vi "Load Config.vi"(8 "error in (no error)":errorcluster, 11 "CurrentInChannel in":refnum<class "CurrentInChannel.lvclass">) -> (0 "error out":errorcluster, 3 "CurrentInChannel out":refnum<class "CurrentInChannel.lvclass">)   [LabVIEW 2020, in "VolatusDAQConfig.lvlib" / "CurrentInChannel.lvclass"]
uses:
  CurrentInChannel.lvclass
  CurrentInChannel.lvclass/CurrentInChannel.ctl
  VolatusConfig/VolatusConfigElement/VolatusConfigElement.lvclass
  lv-cdm/CDM-Config/Config Element/Config Element.lvclass
  C:/dev/lv20CE/relink/lv-volatus/VolatusDAQConfig/DAQmxChannel/DAQmxChannel.lvclass
  C:/dev/lv20CE/relink/lv-volatus/VolatusConfig/Channel/Channel Config.lvclass
  C:/dev/lv20CE/relink/lv-volatus/VolatusConfig/VolatusConfigElement/VolatusConfigElement.lvclass
  C:/dev/lv20CE/relink/lv-volatus/VolatusDAQConfig/CurrentInChannel/CurrentInChannel.lvclass
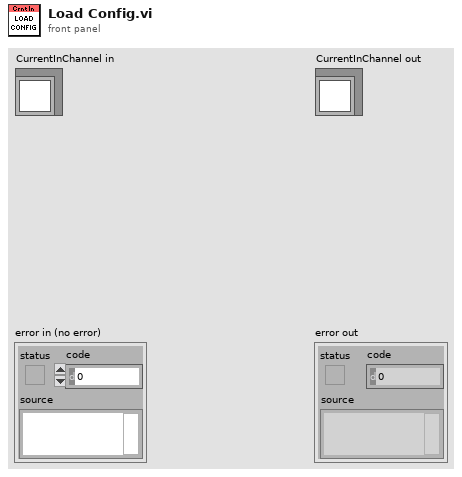
[diagram p1: front panel]
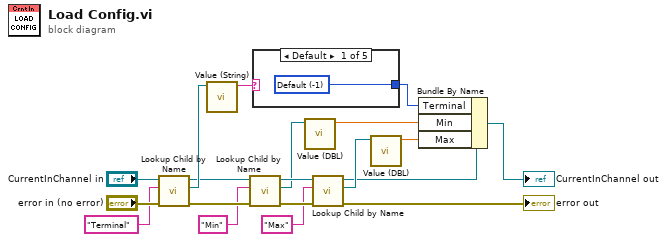
[diagram p0: block diagram]
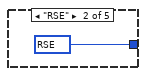
[diagram p2: hidden frame]
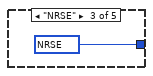
[diagram p3: hidden frame]
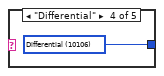
[diagram p4: hidden frame]
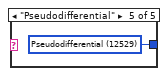
[diagram p5: hidden frame]
diagram:
  n1 = call "Lookup Child by Name.vi"("error in (no error)"="error in (no error)", "Child Name"="Terminal", "VolatusConfigElement in"="CurrentInChannel in") -> ("error out"=w18:errorcluster, "Child"=w17:refnum<class "Config Element.lvclass">, "VolatusConfigElement out"=w13:refnum<class "CurrentInChannel.lvclass">)  [unwired: 5 in, 1 out]
  n2 = call "Value (String).vi"("Config Element in"=w17) -> ("String Value"=w16:string)  [unwired: 9 in, 1 out]
  n3 = call "Lookup Child by Name.vi"("error in (no error)"=w18, "Child Name"="Min", "VolatusConfigElement in"=w13) -> ("error out"=w14:errorcluster, "Child"=w10:refnum<class "Config Element.lvclass">, "VolatusConfigElement out"=w12:refnum<class "CurrentInChannel.lvclass">)  [unwired: 5 in, 1 out]
  n4 = case shown="Default" w16 {
    tunnel: [w20 w21 w22 w23 w24] -> w15
    frame Default {
      w20 = -1 items=["Default"=-1, "RSE"=10083, "NRSE"=10078, "Differential"=10106, "Pseudodifferential"=12529] ("input terminal configuration")
    }
    frame "RSE" {
      w21 = 10083 items=["Default"=-1, "RSE"=10083, "NRSE"=10078, "Differential"=10106, "Pseudodifferential"=12529] ("input terminal configuration")
    }
    frame "NRSE" {
      w22 = 10078 items=["Default"=-1, "RSE"=10083, "NRSE"=10078, "Differential"=10106, "Pseudodifferential"=12529] ("input terminal configuration")
    }
    frame "Differential" {
      w23 = 10106 items=["Default"=-1, "RSE"=10083, "NRSE"=10078, "Differential"=10106, "Pseudodifferential"=12529] ("input terminal configuration")
    }
    frame "Pseudodifferential" {
      w24 = 12529 items=["Default"=-1, "RSE"=10083, "NRSE"=10078, "Differential"=10106, "Pseudodifferential"=12529] ("input terminal configuration")
    }
  }
  n5 = call "Value (DBL).vi"("Config Element in"=w10) -> ("DBL Value"=w9:dbl)  [unwired: 9 in, 1 out]
  n6 = call "Lookup Child by Name.vi"("error in (no error)"=w14, "Child Name"="Max", "VolatusConfigElement in"=w12) -> ("error out"=→"error out":errorcluster, "Child"=w8:refnum<class "Config Element.lvclass">, "VolatusConfigElement out"=w2:refnum<class "CurrentInChannel.lvclass">)  [unwired: 5 in, 1 out]
  n7 = call "Value (DBL).vi"("Config Element in"=w8) -> ("DBL Value"=w7:dbl)  [unwired: 9 in, 1 out]
  n8 = Bundle By Name(cluster=w2, "Terminal"=w15, "Min"=w9, "Max"=w7) -> (→"CurrentInChannel out":refnum<class "CurrentInChannel.lvclass">)
